vi "Create Double Pointer.vi"(8 "error in (no error)":errorcluster, 11 "channel count":u64) -> (0 "error out":errorcluster, 3 "DBL Pointer out":refnum<class "Double Pointer.lvclass">)   [LabVIEW 2017, in "Data Sharing Framework Core.lvlib" / "Data Sharing Framework Engine.lvlib" / "Double Pointer.lvclass"]
uses:
  Double Pointer.lvclass
  C:/Program Files (x86)/National Instruments/LabVIEW 2017/vi.lib/National Instruments/Memory Manager/Classes/Pointer/Memory.Pointer.lvclass
  Double Pointer.lvclass/Double Pointer.ctl
  <vilib>/National Instruments/Memory Manager/Classes/Pointer/Memory.Pointer.lvclass/Memory.Pointer.ctl
  <vilib>/National Instruments/Memory Manager/Classes/Pointer/Memory.Pointer.New.8B.vi
  <vilib>/National Instruments/Memory Manager/Classes/Pointer/Memory.Pointer.Allocate.vi
  <vilib>/National Instruments/Memory Manager/Classes/Pointer/Memory.Pointer.Set Address.vi
  <vilib>/National Instruments/Memory Manager/Classes/Pointer/Memory.Pointer.Set Size.vi
  <vilib>/National Instruments/Memory Manager/Classes/Pointer/Memory.Pointer.Set Allocated.vi
  <vilib>/National Instruments/Memory Manager/Classes/Pointer/Memory.Pointer.lvclass
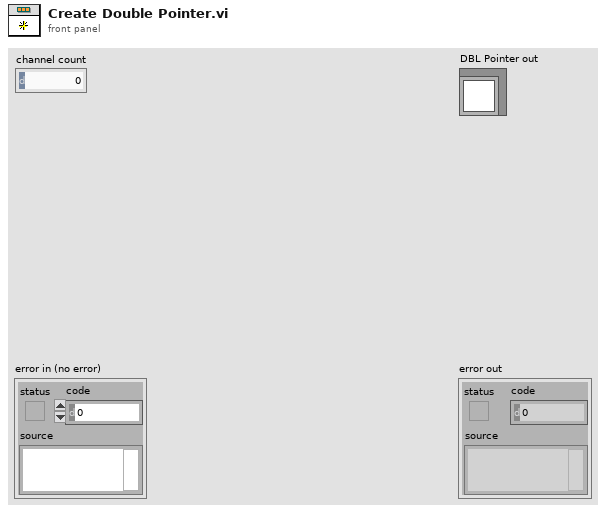
[diagram p1: front panel]
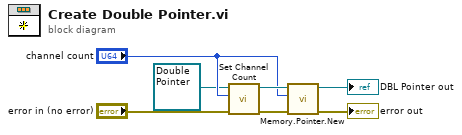
[diagram p0: block diagram]
diagram:
  n1 = call "Set Channel Count.vi"("channel count"="channel count", "DBL Buffer in"=refnum<class "Double Pointer.lvclass"> refnum) -> ("DBL Buffer out"=w6:refnum<class "Double Pointer.lvclass">)  [unwired: 9 in]
  n2 = call-poly <vilib>:"Memory.Pointer.New.vi"("error in (no error)"="error in (no error)", "count (1)"="channel count", "Pointer type"=w6) -> ("error out"=→"error out":errorcluster, "Pointer"=→"DBL Pointer out":refnum<class "Double Pointer.lvclass">)  [unwired: 7 in]
